vi "testGenData.vi"() -> (3 "Array":u32[][](array[numeric]))   [LabVIEW 2024]
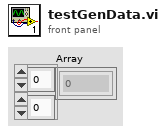
[diagram p1: front panel]
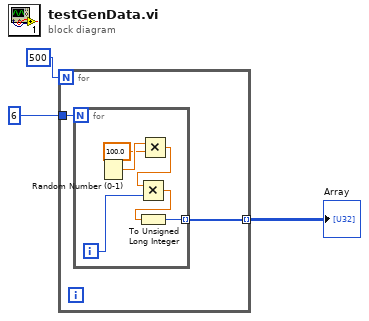
[diagram p0: block diagram]
diagram:
  n1 = for {
    N: 500 -> [_]
    tunnel: 6 -> [w5]
    tunnel: [w4] -> w3 mode=indexing
    n2 = for {
      N: w5 -> [_]
      tunnel: [w6] -> w4 mode=indexing
      i -> [w8]
      n3 = Random Number (0-1)() -> (number: 0 to 1=w11:dbl)
      n4 = Multiply(x=w11, y=100.0) -> (x*y=w9:dbl)
      n5 = Multiply(x=w9, y=w8) -> (x*y=w7:dbl)
      n6 = To Unsigned Long Integer(number=w7) -> (unsigned 32bit integer=w6:u32)
    }
  }
  "Array" <- w3
